vi "START!.vi"() -> ()   [LabVIEW 2014]
doc: "Launches all the software required for data acquisition."
uses:
  Start all VIs Globals.vi
panel:
  out "Starting Module Number:":u32(slide) scale=0.0..10.0
  out "Status":string="Ready"
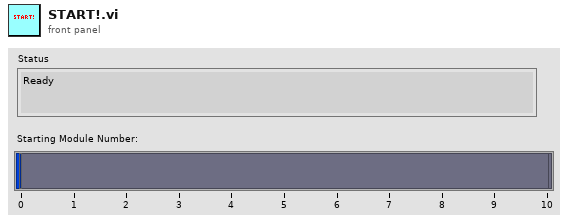
[diagram p1: front panel]
types:
  T1 = cluster{"VI Name":string, "Location":enum16{"TIRF Lock", "Camera & Acquisition VIs", "Stage Control", "Shutter Control"}, "Run?":bool, "Minimized?":bool, "Subdirectory (w trailing \"/\")":string}[]
  T2 = cluster{"Shutter Control":path, "Stage Control":path, "Camera & Acquisition VIs":path, "TIRF Lock":path}
  T3 = enum32{"Invalid", "Standard", "Closed", "Hidden", "Minimized", "Maximized"}
  T4 = enum16{"TIRF Lock", "Camera & Acquisition VIs", "Stage Control", "Shutter Control"}
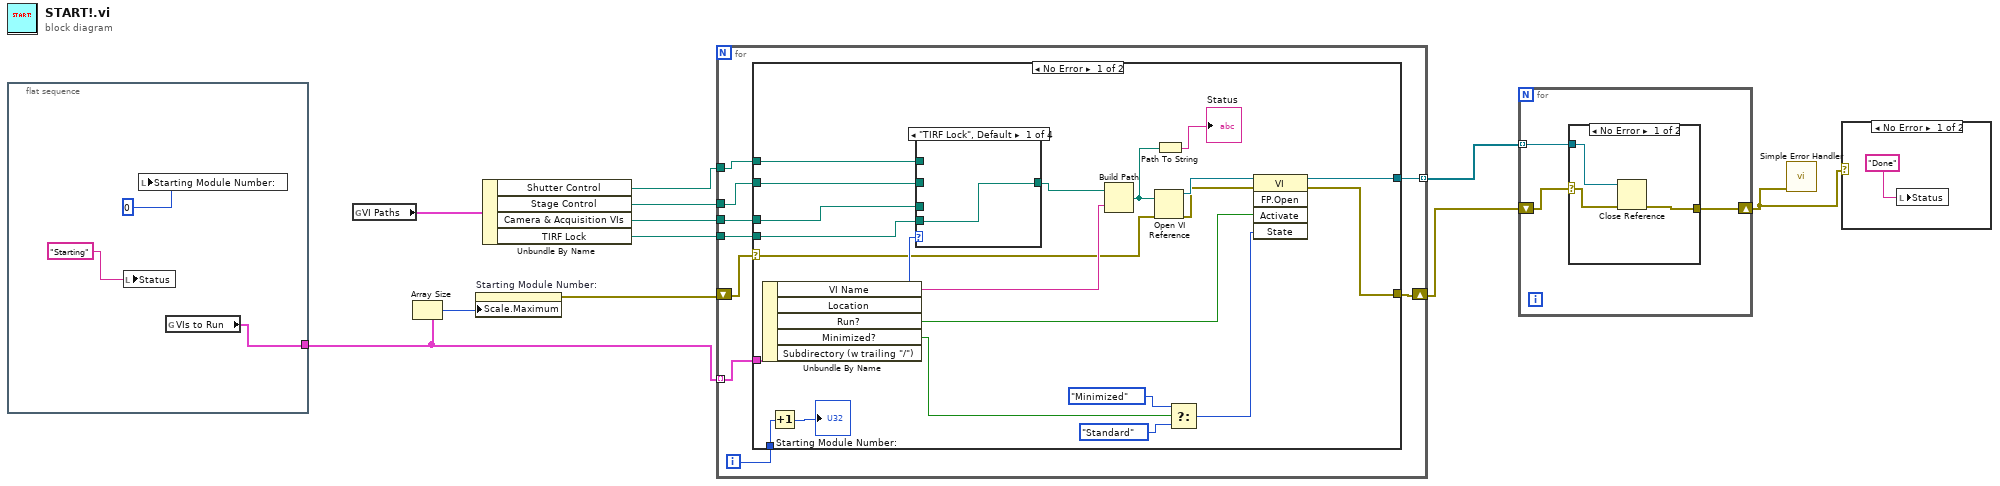
[diagram p0: block diagram]
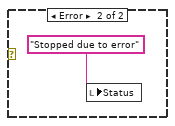
[diagram p2: hidden frame]
diagram:
  n1 = flat-sequence {
    tunnel: [w14] -> w1
    frame #0 {
      n2 = local write "Status"("Starting") -> ()
      n3 = local write "Starting Module Number:"(0) -> ()
      n4 = global read "Start all VIs Globals.vi" "VIs to Run"() -> (w14:T1)
    }
  }
  n5 = global read "Start all VIs Globals.vi" "VI Paths"() -> (w11:T2)
  n6 = Array Size(array=w1) -> (size(s)=w2:i32)
  n7 = property on="Starting Module Number:" class="Slide (strict)"("Scale.Maximum"=w2) -> (error out=w3:errorcluster)  [unwired: 2 in, 1 out]
  n8 = Unbundle By Name(w11) -> ("Shutter Control"=w10:path, "Stage Control"=w9:path, "Camera & Acquisition VIs"=w8:path, "TIRF Lock"=w7:path)
  n9 = for {
    tunnel: w10 -> [w22]
    tunnel: w9 -> [w21]
    tunnel: w8 -> [w20]
    tunnel: w7 -> [w19]
    tunnel: w1 -> [w23] mode=indexing
    tunnel: [w18] -> w6 mode=indexing
    shift-right: [w17] -> w5
    shift-left: w3 -> [w16]
    i -> [w15]
    n10 = case shown="No Error" w16 {
      selector: w16 -> [w28 w50]
      tunnel: w23 -> [w45 _]
      tunnel: w22 -> [w43 _]
      tunnel: w21 -> [w42 _]
      tunnel: w20 -> [w41 _]
      tunnel: w19 -> [w40 _]
      tunnel: [w30 _] -> w18
      tunnel: [w29 w50] -> w17
      tunnel: w15 -> [w26 _]
      frame No Error {
        n11 = Unbundle By Name(w45) -> ("VI Name"=w38:string, "Location"=w44:T4, "Run?"=w35:bool, "Minimized?"=w32:bool)  [unwired: 1 out]
        n12 = Increment(x=w26) -> (x+1=→"Starting Module Number:":i32)
        n13 = case shown="\"TIRF Lock\", Default" w44 {
          tunnel: w43 -> [_ _ _ w49]
          tunnel: w42 -> [_ _ w48 _]
          tunnel: w41 -> [_ w47 _ _]
          tunnel: w40 -> [w46 _ _ _]
          tunnel: [w46 w47 w48 w49] -> w39
          frame "TIRF Lock", Default {
          }
          frame "Camera & Acquisition VIs" {
          }
          frame "Stage Control" {
          }
          frame "Shutter Control" {
          }
        }
        n14 = Build Path(base path=w39, name or relative path=w38) -> (appended path=w24:path)
        n15 = Open VI Reference(vi path=w24, error in (no error)=w28) -> (vi reference=w37:refnum<vi>, error out=w36:errorcluster)  [unwired: 4 out]
        n16 = Path To String(path=w24) -> (string=→"Status":string)
        n17 = Select(t=T3."Minimized" ("State"), s=w32, f=T3."Standard" ("State")) -> (s? t:f=w31:T3)
        n18 = invoke class="VI" method="FP.Open"(reference=w37, error in=w36, "Activate"=w35, "State"=w31) -> (reference out=w30:refnum<vi>, error out=w29:errorcluster)  [unwired: 1 in, 3 out]
      }
      frame Error {
      }
    }
  }
  n19 = for {
    tunnel: w6 -> [w53] mode=indexing
    shift-right: [w52] -> w4
    shift-left: w5 -> [w51]
    n20 = case shown="No Error" w51 {
      selector: w51 -> [w56 w57]
      tunnel: w53 -> [w55 _]
      tunnel: [w54 w57] -> w52
      frame No Error {
        n21 = Close Reference(reference=w55, error in (no error)=w56) -> (error out=w54:errorcluster)
      }
      frame Error {
      }
    }
  }
  n22 = call <vilib>:"Simple Error Handler.vi"("error in (no error)"=w4) -> ()  [unwired: 4 in, 5 out]
  n23 = case shown="No Error" w4 {
    frame No Error {
      n24 = local write "Status"("Done") -> ()
    }
    frame Error {
      n25 = local write "Status"("Stopped due to error") -> ()
    }
  }
